vi "Initialize Configuration.vi"(8 "error in (no error)":errorcluster, 11 "Instrument in":refnum<class "Instrument.lvclass">) -> (0 "error out":errorcluster, 3 "Instrument out":refnum<class "Instrument.lvclass">)   [LabVIEW 2019, in "Instrument.lvlib" / "Instrument.lvclass"]
uses:
  Instrument.lvclass
  Instrument.lvclass/Instrument.ctl
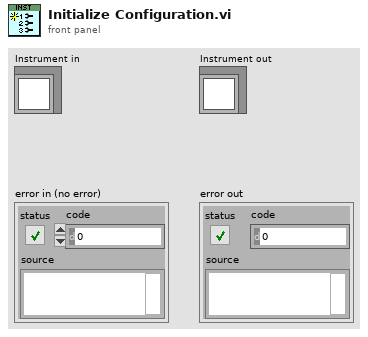
[diagram p1: front panel]
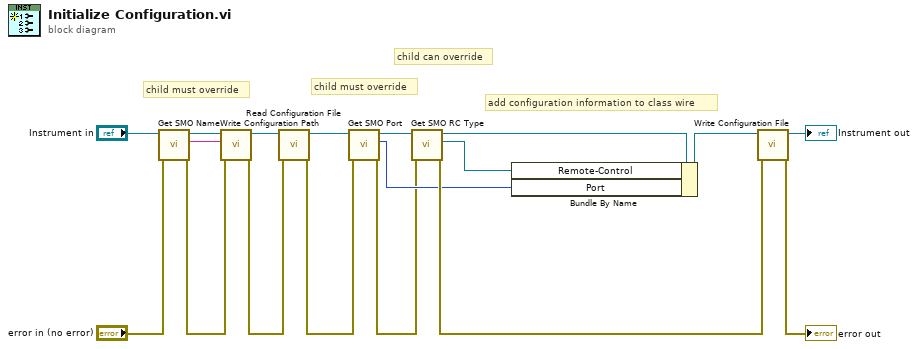
[diagram p0: block diagram]
diagram:
  # "child can override"
  # "child must override"
  # "child must override"
  # "add configuration information to class wire"
  n1 = call-dynamic "Get SMO Name.vi"("error in (no error)"="error in (no error)", "Instrument in"="Instrument in") -> ("error out"=w5:errorcluster, "SMO Name"=w14:string, "Instrument out"=w6:refnum<class "Instrument.lvclass">)  [unwired: 7 in]
  n2 = call "Write Configuration Path.vi"("error in (no error)"=w5, "name or relative path"=w14, "Instrument in"=w6) -> ("error out"=w12:errorcluster, "Instrument out"=w11:refnum<class "Instrument.lvclass">)  [unwired: 7 in]
  n3 = call-dynamic "Read Configuration File.vi"("error in (no error)"=w12, "Instrument in"=w11) -> ("error out"=w1:errorcluster, "Instrument out"=w13:refnum<class "Instrument.lvclass">)  [unwired: 8 in]
  n4 = call-dynamic "Get SMO Port.vi"("error in (no error)"=w1, "Instrument in"=w13) -> ("error out"=w8:errorcluster, "Port"=w9:u16, "Instrument out"=w7:refnum<class "Instrument.lvclass">)  [unwired: 7 in]
  n5 = call-dynamic "Get SMO RC Type.vi"("error in (no error)"=w8, "Instrument in"=w7) -> ("error out"=w16:errorcluster, "RemoteControl"=w2:refnum<class "RemoteControl.lvclass">, "Instrument out"=w10:refnum<class "Instrument.lvclass">)  [unwired: 7 in]
  n6 = Bundle By Name(cluster=w10, "Remote-Control"=w2, "Port"=w9) -> (w18:refnum<class "Instrument.lvclass">)
  n7 = call-dynamic "Write Configuration File.vi"("error in (no error)"=w16, "Instrument in"=w18) -> ("error out"=→"error out":errorcluster, "Instrument out"=→"Instrument out":refnum<class "Instrument.lvclass">)  [unwired: 8 in]
